vi "initialise.vi"(8 "error in (no error)":errorcluster, 11 "YK090623DAQmxAnalogDetector in":refnum<class "DetectorYK090623DAQmxAnalog.lvclass">) -> (0 "error out":errorcluster, 3 "YK090623DAQmxAnalogDetector out":refnum<class "DetectorYK090623DAQmxAnalog.lvclass">)   [LabVIEW 2010, in "DetectorYK090623DAQmxAnalog.lvclass"]
doc: "The dynamic dispatch-version of this VI initalises the plug-in object by allocating and initalising any dynamic resources need."
uses:
  DetectorYK090623DAQmxAnalog.lvclass
  GenericDetector/GenericDetector/GenericDetector.lvclass
  DetectorYK090623DAQmxAnalog.lvclass/DetectorYK090623DAQmxAnalog.ctl
  AnalogOut/AnalogOutDL101207DAQmx/AnalogOutDL101207DAQmx/AnalogOutDL101207DAQmx.lvclass
  common/classes/ErrorController/ErrorController/class_data.vi
  common/classes/ErrorController/ErrorController/ErrorController.lvclass
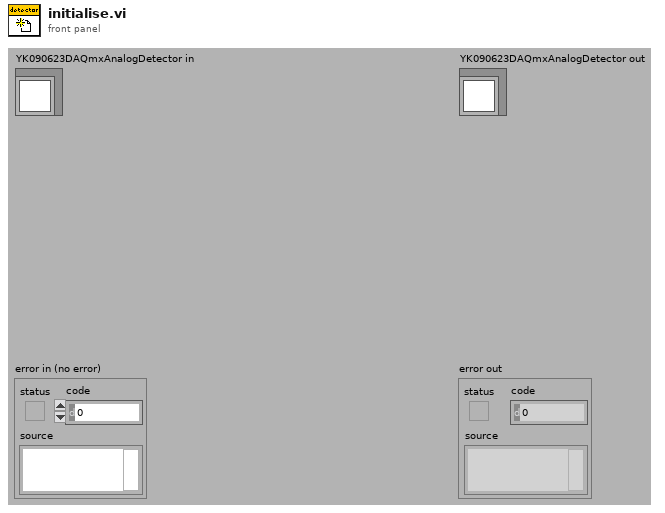
[diagram p1: front panel]
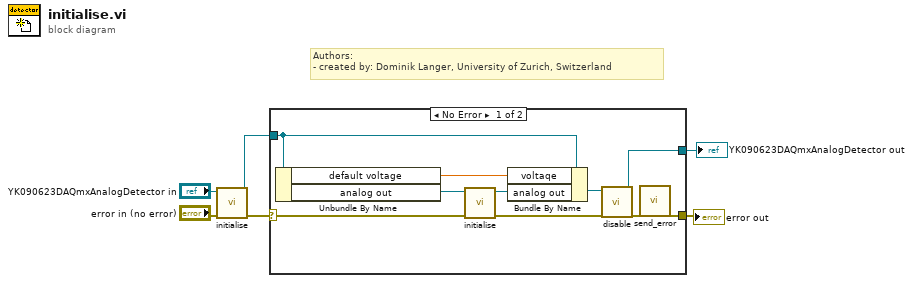
[diagram p0: block diagram]
diagram:
  # "Authors: \n- created by: Dominik Langer, University of Zurich, Switzerland"
  n1 = call-parent "initialise.vi"("error in (no error)"="error in (no error)", "GenericPlugin in"="YK090623DAQmxAnalogDetector in") -> ("error out"=w4:errorcluster, "GenericPlugin out"=w3:refnum<class "DetectorYK090623DAQmxAnalog.lvclass">)  [unwired: 8 out]
  n2 = case shown="No Error" w4 {
    selector: w4 -> [w16 w17]
    tunnel: w3 -> [w14 w18]
    tunnel: [w7 w17] -> w2
    tunnel: [w9 w18] -> w1
    frame No Error {
      n3 = Unbundle By Name(w14) -> ("default voltage"=w13:dbl[unit], "analog out"=w15:refnum<class "AnalogOutDL101207DAQmx.lvclass">)
      n4 = call-dynamic "initialise.vi"("error in (no error)"=w16, "DAQmxAnalogOut in"=w15) -> ("error out"=w11:errorcluster, "DAQmxAnalogOut out"=w12:refnum<class "AnalogOutDL101207DAQmx.lvclass">)  [unwired: 8 out]
      n5 = Bundle By Name(cluster=w14, "voltaqe"=w13, "analog out"=w12) -> (w10:refnum<class "DetectorYK090623DAQmxAnalog.lvclass">)
      n6 = call-dynamic "disable.vi"("error in (no error)"=w11, "GenericEmissionSensor in"=w10) -> ("error out"=w8:errorcluster, "GenericEmissionSensor out"=w9:refnum<class "DetectorYK090623DAQmxAnalog.lvclass">)  [unwired: 8 out]
      n7 = call "send_error.vi"("error in (no error)"=w8) -> ("error out"=w7:errorcluster)  [unwired: 10 in]
    }
    frame Error {
    }
  }
  "error out" <- w2
  "YK090623DAQmxAnalogDetector out" <- w1
